vi "Image Array User Event_Algo.vi"(8 "error in (no error)":errorcluster, 10 "Image Array":T1[](array[typedef]), 11 "Algorithm in":refnum<class "Algorithm.lvclass">) -> (0 "error out":errorcluster, 3 "Algorithm out":refnum<class "Algorithm.lvclass">)   [LabVIEW 2015]
uses:
  FrameworkOverrides/Algorithm.lvclass
  <vilib>/vision/Image Controls.llb/IMAQ Image.ctl
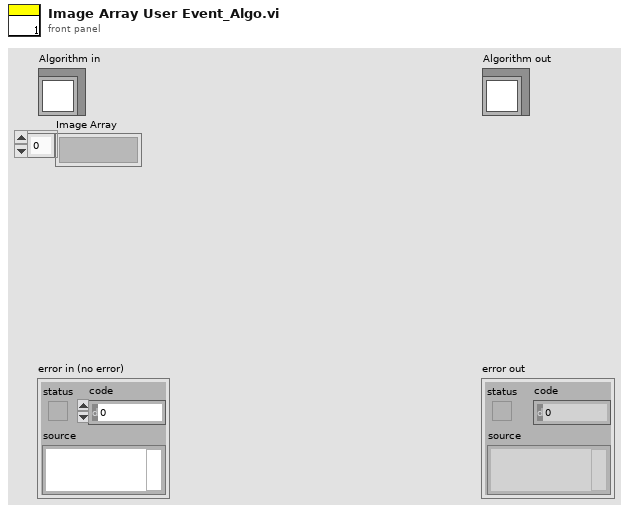
[diagram p1: front panel]
types:
  T1 = typedef "IMAQ Image.ctl" = refnum<image>
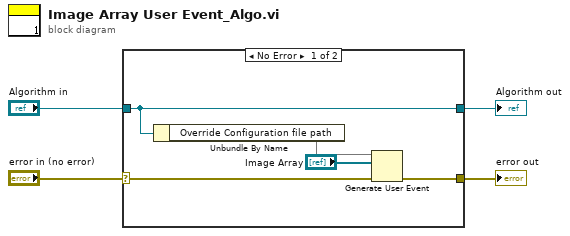
[diagram p0: block diagram]
diagram:
  n1 = case shown="No Error" "error in (no error)" {
    selector: "error in (no error)" -> [w6 w11]
    tunnel: [w5 w11] -> w3
    tunnel: [w9 w10] -> w1
    tunnel: "Algorithm in" -> [w9 w10]
    frame No Error {
      n2 = Unbundle By Name(w9) -> ("Override Configuration file path"=w8)
      n3 = Generate User Event(user event=w8, event data cluster="Image Array", error in=w6) -> (error out=w5:errorcluster)  [unwired: 1 in, 1 out]
    }
    frame Error {
    }
  }
  "error out" <- w3
  "Algorithm out" <- w1
